vi "Load New Bitfile.vi"(7 "Group":bool, 8 "error in (no error)":errorcluster, 10 "NewVal":path, 11 "Item Ref in":T1 format="%.0x") -> (0 "error out":errorcluster, 3 "Section Ref out":T1 format="%.0x")   [LabVIEW 2018, in "FPGA Addon System Explorer.lvlib"]
uses:
  FPGA Addon System Explorer.lvlib
  <vilib>/NI Veristand/Custom Device API/Custom Device Item Ref.ctl
  Addon Shared/Types/FG Action.ctl
  Addon Shared/SubVIs/Constants.vi
  <vilib>/NI Veristand/Custom Device Tools/Custom Device Utility Library/NI VeriStand - Search for Item by GUID.vi
  <vilib>/NI/NI VeriStand Advanced SysDef API/SysDef API/SysDef.Property.Get.vi
  <vilib>/NI/NI VeriStand Advanced SysDef API/_SubVIs/SysDef.Property.Get.Variant.vi
  <vilib>/NI/NI VeriStand Advanced SysDef API/SysDef API/SysDef.Property.Set.vi
  <vilib>/NI/NI VeriStand Advanced SysDef API/_SubVIs/SysDef.Property.Set.Variant.vi
  Addon Shared/FPGA Addon Shared.lvlib
  <vilib>/NI Veristand/Custom Device API/Custom Device API.lvlib
  <vilib>/NI Veristand/Custom Device Tools/Custom Device Utility Library/Custom Device Utility Library.lvlib
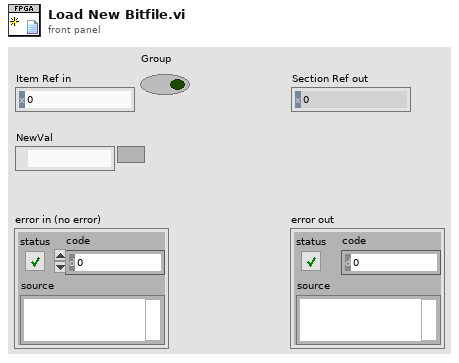
[diagram p1: front panel]
types:
  T1 = typedef "Custom Device API.lvlib/Custom Device Item Ref.ctl" = u64
  T2 = typedef "FPGA Addon Shared.lvlib/FG Action.ctl" = enum8{"GET", "SET"}
  T3 = typedef "Fifo_DMA_Config.ctl" = cluster{"Name":string, "Depth":u32, "Write? (Deprecated:Use Implementation)":bool, "Physical Channel":u32, "Base Address":u32, "Data Width":u32, "Data Type":T4, "FXP Properties":variant, "Write Window Address":u32, "Implementation":T5, "Control Set":u32}
  T4 = typedef "niFpgaDataTypeControl.ctl" = enum32{"Boolean", "I8", "I16", "I32", "I64", "U8", "U16", "U32", "U64", "FXP", "CustomControl", "SGL"}
  T5 = typedef "niFpgaDmaChannelImplementation.ctl" = enum16{"niFpgaTargetToHost", "niFpgaHostToTarget", "niFpgaPeerToPeerWriter", "niFpgaPeerToPeerReader", "niCoreTargetToHost", "niCoreHostToTarget"}
  T6 = typedef "niFpgaBitfileStructure_VI.ctl" = cluster{"Name":string, "RegisterMap":T7[], "Icon":T12}
  T7 = typedef "nirviControlStructure.ctl" = cluster{"Name":string, "Hidden":bool, "Indicator":bool, "Flattened Type":string, "Grouping":cluster{"Grouped":bool, "Member Names":string[], "Member IDs":u32[]}, "Address":u32, "Size":u32, "Class":u32, "Internal":bool, "Typedef":T8, "ID":u32, "Bidirectional":bool, "Synchronous":bool, "Mechanical Action":T9, "Sub Controls":T10[], "Access May Timeout":bool, "Register Node":bool}
  T8 = typedef "nirviTypdefDescription.ctl" = cluster{"Typedef":bool, "Path":path}
  T9 = typedef "nirviMechanicalAction.ctl" = enum8{"Switch When Pressed", "Switch When Released", "Switch Until Released", "Latch When Pressed", "Latch When Released", "Latch Until Released"}
  T10 = typedef "nirviSubControlStructure.ctl" = cluster{"Name":string, "flattened Type":string, "Cluster Information":T11, "Typedef":T8}
  T11 = typedef "nirviClusterElementControl.ctl" = cluster{"Name Hierarchy":string[], "Item Order":u32[]}
  T12 = typedef "imagedata.ctl" = cluster{"image type":i32, "image depth":i32, "image":u8[], "mask":u8[], "colors":u32[], "Rectangle":cluster{"left":i16, "top":i16, "right":i16, "bottom":i16}}
  T13 = typedef "FPGA Addon Shared.lvlib/Register Information.ctl" = cluster{"Name":string, "Data Type":T14, "Default Value":variant}
  T14 = typedef "FPGA Addon Shared.lvlib/Data Type.ctl" = enum8{"<Null>", "I8", "I16", "I32", "I64", "U8", "U16", "U32", "U64", "SGL", "Boolean", "Analog PWM In Settings", "Analog PWM In", "Digital PWM In Settings", "Digital PWM In", "Digital PWM Out", "Sine Out", "FXP+/-24.5", "FXP+/-16.5", "FXP+/-32.8", "FXP+/-64.32", "FXP+/-16.7", "FXP+/-20.5", "FXP+/-27.5", "FXP+/-32.16", "FXP+16.3", "FXP+18.3", "Digital Static In", "Digital Static Out", "Digital Static In Settings", "Digital WSS Out", "Quad Encoder Settings", "Quad Encoder In", "Group"}
  T15 = typedef "FPGA Addon Shared.lvlib/DMA Information.ctl" = cluster{"Name":string, "Data Type":T14}
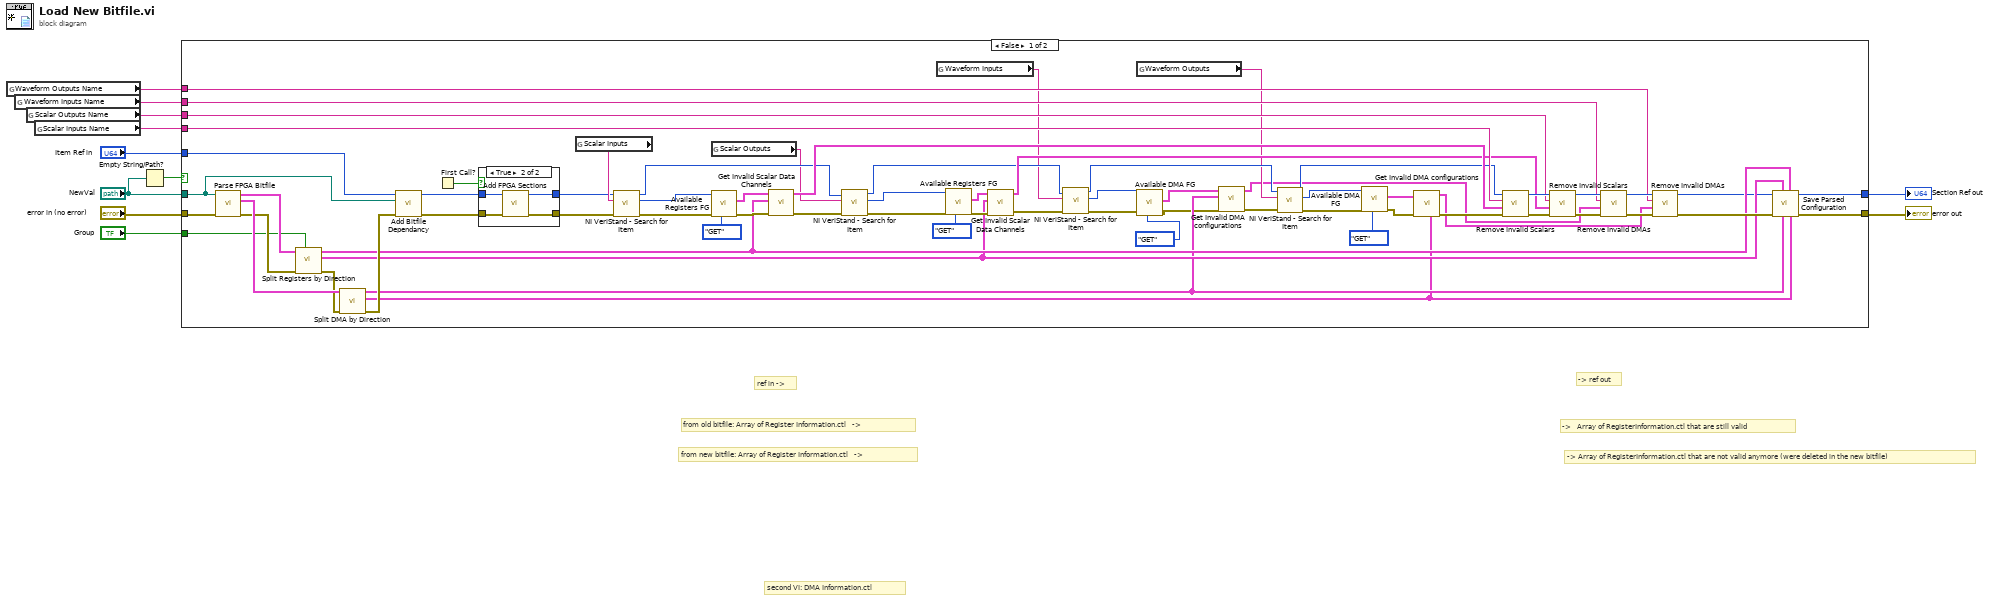
[diagram p0: block diagram]
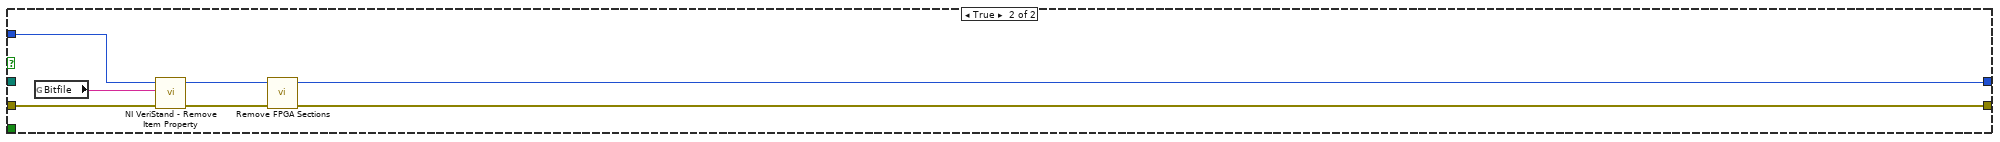
[diagram p3: hidden frame]
diagram:
  # "second VI: DMA Information.ctl"
  # "-> Array of RegisterInformation.ctl that are not valid anymore (were deleted in the new bitfile)"
  # "-> ref out"
  # "ref in ->"
  # "->   Array of RegisterInformation.ctl that are still valid"
  # "from new bitfile: Array of Register Information.ctl   ->"
  # "from old bitfile: Array of Register Information.ctl   ->"
  n1 = global read "Constants.vi" "Waveform Outputs Name"() -> (w8:string)
  n2 = global read "Constants.vi" "Waveform Inputs Name"() -> (w9:string)
  n3 = global read "Constants.vi" "Scalar Outputs Name"() -> (w10:string)
  n4 = global read "Constants.vi" "Scalar Inputs Name"() -> (w11:string)
  n5 = Empty String/Path?(string/path="NewVal") -> (empty?=w5:bool)
  n6 = case shown="False" w5 {
    tunnel: "NewVal" -> [w72 _]
    tunnel: "error in (no error)" -> [w77 w85]
    tunnel: w11 -> [w48 _]
    tunnel: w10 -> [w51 _]
    tunnel: w9 -> [w43 _]
    tunnel: w8 -> [w39 _]
    tunnel: [w74 w90] -> w7
    tunnel: [w73 w89] -> w6
    tunnel: "Item Ref in" -> [w71 w87]
    tunnel: "Group" -> [w67 _]
    frame False {
      n7 = call "Parse FPGA Bitfile.vi"("error in (no error)"=w77, "Path"=w72) -> ("error out"=w70:errorcluster, "DMA configuration array"=w76:T3[], "vi info"=w75:T6)  [unwired: 7 in]
      n8 = call "Split Registers by Direction.vi"("Group"=w67, "error in"=w70, "vi info"=w75) -> ("error out"=w69:errorcluster, "Controls"=w45:T13[], "Indicator"=w54:T13[])  [unwired: 6 in]
      n9 = call "Split DMA by Direction.vi"("error in"=w69, "DMA configuration array"=w76) -> ("error out"=w68:errorcluster, "HostToTarget"=w38:T15[], "TargetToHost"=w41:T15[])  [unwired: 7 in]
      n10 = call "Add Bitfile Dependancy.vi"("error in (no error)"=w68, "Path"=w72, "Item Ref in"=w71) -> ("error out"=w27:errorcluster, "Item Ref out"=w28:T1)  [unwired: 7 in]
      n11 = First Call?() -> (First Call?: T/F=w24:bool)
      n12 = case shown="True" w24 {
        tunnel: w28 -> [w79 w83]
        tunnel: w27 -> [w78 w82]
        tunnel: [w78 w81] -> w26
        tunnel: [w79 w80] -> w25
        frame False {
        }
        frame True {
          n13 = call "Add FPGA Sections.vi"("error in (no error)"=w82, "Node Ptr"=w83) -> ("error out"=w81:errorcluster, "Parent Ref out"=w80:T1)  [unwired: 8 in]
        }
      }
      n14 = global read "Constants.vi" "Scalar Inputs"() -> (w32:string)
      n15 = call-poly <vilib>:"NI VeriStand - Search for Item.vi"("error in"=w26, "Item GUID"=w32, "Section Ref in"=w25) -> ("error out"=w59:errorcluster, "Item Ref"=w58:T1, "Section Ref out"=w49:T1)  [unwired: 5 in, 1 out]
      n16 = global read "Constants.vi" "Scalar Outputs"() -> (w31:string)
      n17 = call "Available Registers FG.vi"("Action"=FG_Action."GET", "error in (no error)"=w59, "Item Ref"=w58) -> ("error out"=w56:errorcluster, "Available Registers"=w55:T13[])  [unwired: 6 in, 1 out]
      n18 = call "Get Invalid Scalar Data Channels.vi"("error in (no error)"=w56, "new bitfile scalar channels"=w54, "old bitfile scalar channels"=w55) -> ("error out"=w52:errorcluster, "invalid scalar data channels"=w53:T13[])  [unwired: 6 in, 1 out]
      n19 = call-poly <vilib>:"NI VeriStand - Search for Item.vi"("Item GUID"=w31, "Section Ref in"=w49) -> ("Item Ref"=w50:T1, "Section Ref out"=w33:T1)  [unwired: 6 in, 2 out]
      n20 = global read "Constants.vi" "Waveform Inputs"() -> (w30:string)
      n21 = call "Available Registers FG.vi"("Action"=FG_Action."GET", "Item Ref"=w50) -> ("Available Registers"=w46:T13[])  [unwired: 7 in, 2 out]
      n22 = call "Get Invalid Scalar Data Channels.vi"("error in (no error)"=w52, "new bitfile scalar channels"=w45, "old bitfile scalar channels"=w46) -> ("error out"=w42:errorcluster, "invalid scalar data channels"=w44:T13[])  [unwired: 6 in, 1 out]
      n23 = call-poly <vilib>:"NI VeriStand - Search for Item.vi"("error in"=w42, "Item GUID"=w30, "Section Ref in"=w33) -> ("error out"=w22:errorcluster, "Item Ref"=w23:T1, "Section Ref out"=w35:T1)  [unwired: 5 in, 1 out]
      n24 = global read "Constants.vi" "Waveform Outputs"() -> (w29:string)
      n25 = call "Available DMA FG.vi"("Action"=FG_Action."GET", "error in (no error)"=w22, "Item Ref"=w23) -> ("error out"=w21:errorcluster, "Available DMA"=w20:T15[])  [unwired: 6 in, 1 out]
      n26 = call "Get Invalid DMA configurations.vi"("error in (no error)"=w21, "new bitfile dma configuration"=w41, "old bitfile dma configuration"=w20) -> ("error out"=w40:errorcluster, "invalid dma configurations"=w18:T15[])  [unwired: 6 in, 1 out]
      n27 = call-poly <vilib>:"NI VeriStand - Search for Item.vi"("error in"=w40, "Item GUID"=w29, "Section Ref in"=w35) -> ("error out"=w16:errorcluster, "Item Ref"=w17:T1, "Section Ref out"=w34:T1)  [unwired: 5 in, 1 out]
      n28 = call "Available DMA FG.vi"("Action"=FG_Action."GET", "error in (no error)"=w16, "Item Ref"=w17) -> ("error out"=w14:errorcluster, "Available DMA"=w13:T15[])  [unwired: 6 in, 1 out]
      n29 = call "Get Invalid DMA configurations.vi"("error in (no error)"=w14, "new bitfile dma configuration"=w38, "old bitfile dma configuration"=w13) -> ("error out"=w37:errorcluster, "invalid dma configurations"=w12:T15[])  [unwired: 6 in, 1 out]
      n30 = call "Remove Invalid Scalars.vi"("error in (no error)"=w37, "Invalid"=w53, "Section Name"=w48, "Item Ref in"=w34) -> ("error out"=w66:errorcluster, "Item Ref out"=w62:T1)  [unwired: 6 in]
      n31 = call "Remove Invalid Scalars.vi"("error in (no error)"=w66, "Invalid"=w44, "Section Name"=w51, "Item Ref in"=w62) -> ("error out"=w65:errorcluster, "Item Ref out"=w61:T1)  [unwired: 6 in]
      n32 = call "Remove Invalid DMAs.vi"("error in (no error)"=w65, "invalid"=w18, "Section Name"=w43, "Item Ref in"=w61) -> ("error out"=w64:errorcluster, "Item Ref out"=w60:T1)  [unwired: 6 in]
      n33 = call "Remove Invalid DMAs.vi"("error in (no error)"=w64, "invalid"=w12, "Section Name"=w39, "Item Ref in"=w60) -> ("error out"=w63:errorcluster, "Item Ref out"=w36:T1)  [unwired: 6 in]
      n34 = call "Save Parsed Configuration.vi"("HostToTarget DMAs"=w38, "Indicators"=w54, "TargetToHost DMAs"=w41, "Controls"=w45, "error in (no error)"=w63, "Parent Ref in"=w36) -> ("error out"=w74:errorcluster, "Section Ref out"=w73:T1)  [unwired: 4 in]
    }
    frame True {
      n35 = global read "Constants.vi" "Bitfile"() -> (w88:string)
      n36 = call <vilib>:"NI VeriStand - Remove Item Property.vi"("error in (no error)"=w85, "Property Name"=w88, "Item Ref in"=w87) -> ("error out"=w84:errorcluster, "Item Ref out"=w86:T1)  [unwired: 6 in, 1 out]
      n37 = call "Remove FPGA Sections.vi"("error in (no error)"=w84, "Item Ref in"=w86) -> ("error out"=w90:errorcluster, "Item Ref out"=w89:T1)  [unwired: 8 in]
    }
  }
  "error out" <- w7
  "Section Ref out" <- w6
